vi "Configure Port.vi"(0 "UART Driver in":refnum<class "UART Driver.lvclass">, 1 "Controller Number":u8, 5 "Configuration Parameters":T1={"Baud"=4, "Character Length"=8, "Stop Bits"=enum."1.0", "Parity"=enum."None", "Character Spacing (ticks)"=1}, 11 "error in":errorcluster) -> (4 "UART Driver out":refnum<class "UART Driver.lvclass">, 15 "error out":errorcluster)   [LabVIEW 2013, in "UART_Host_Driver.lvlib" / "UART Driver.lvclass"]
doc: "Initalize the UART port specificed by the RIO Device Name to the specified settings.\n\nMust call UART Initialize.vi, prior to calling UART Configure Port.vi.\n\nNote: Port Number 255 means to transmit to all of the ports configured in the UART Initialize.vi."
uses:
  UART Driver.lvclass
  Typedefs/Configuration Parameters.ctl
  FPGA/UART/StopBits.ctl
  FPGA/UART/Parity.ctl
  FPGA/UART/UART_Firmware.lvlib
  UART_Host_Driver.lvlib
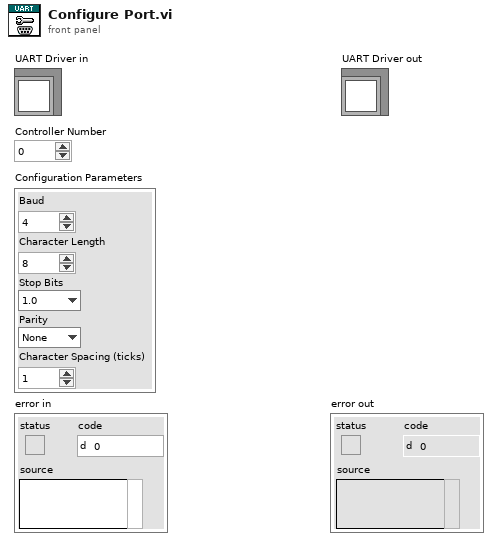
[diagram p1: front panel]
types:
  T1 = typedef "UART_Host_Driver.lvlib/Configuration Parameters.ctl" = cluster{"Baud":u32, "Character Length":u8, "Stop Bits":T2, "Parity":T3, "Character Spacing (ticks)":u32}
  T2 = typedef "UART_Firmware.lvlib/StopBits.ctl" = enum8{"1.0", "1.5", "2.0"}
  T3 = typedef "UART_Firmware.lvlib/Parity.ctl" = enum8{"None", "Even", "Odd"}
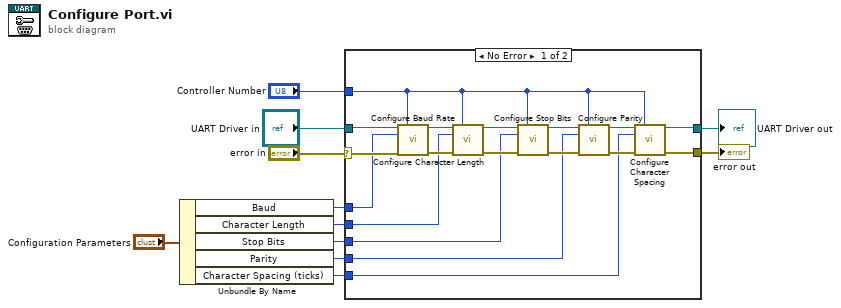
[diagram p0: block diagram]
diagram:
  n1 = Unbundle By Name("Configuration Parameters") -> ("Baud"=w5:u32, "Character Length"=w4:u8, "Stop Bits"=w3:T2, "Parity"=w2:T3, "Character Spacing (ticks)"=w1:u32)
  n2 = case shown="No Error" "error in" {
    selector: "error in" -> [w28 w31]
    tunnel: [w17 w31] -> w10
    tunnel: [w20 w30] -> w7
    tunnel: "UART Driver in" -> [w29 w30]
    tunnel: w5 -> [w16 _]
    tunnel: w4 -> [w15 _]
    tunnel: w3 -> [w14 _]
    tunnel: "Controller Number" -> [w19 _]
    tunnel: w2 -> [w13 _]
    tunnel: w1 -> [w12 _]
    frame No Error {
      n3 = call-dynamic "Configure Baud Rate.vi"("UART Driver in"=w29, "Controller Number"=w19, "Baud Rate"=w16, "error in"=w28) -> ("UART Driver out"=w27:refnum<class "UART Driver.lvclass">, "error out"=w26:errorcluster)  [unwired: 9 in, 1 out]
      n4 = call-dynamic "Configure Character Length.vi"("UART Driver in"=w27, "Controller Number"=w19, "Character Length"=w15, "error in"=w26) -> ("UART Driver out"=w24:refnum<class "UART Driver.lvclass">, "error out"=w23:errorcluster)  [unwired: 9 in, 1 out]
      n5 = call-dynamic "Configure Stop Bits.vi"("UART Driver in"=w24, "Controller Number"=w19, "Stop Bits"=w14, "error in"=w23) -> ("UART Driver out"=w25:refnum<class "UART Driver.lvclass">, "error out"=w22:errorcluster)  [unwired: 9 in, 1 out]
      n6 = call-dynamic "Configure Parity.vi"("UART Driver in"=w25, "Controller Number"=w19, "Parity"=w13, "error in"=w22) -> ("UART Driver out"=w21:refnum<class "UART Driver.lvclass">, "error out"=w18:errorcluster)  [unwired: 9 in, 1 out]
      n7 = call-dynamic "Configure Character Spacing.vi"("UART Driver in"=w21, "Controller Number"=w19, "Spacing (ticks)"=w12, "error in"=w18) -> ("UART Driver out"=w20:refnum<class "UART Driver.lvclass">, "error out"=w17:errorcluster)  [unwired: 9 in, 1 out]
    }
    frame Error {
    }
  }
  "error out" <- w10
  "UART Driver out" <- w7
